vi "Init Sync Stuff.vi"(8 "error in (no error)":errorcluster, 10 "Ambient Light Bricklet in":refnum<class "Ambient Light Bricklet.lvclass">) -> (0 "error out":errorcluster, 2 "Ambient Light Bricklet out":refnum<class "Ambient Light Bricklet.lvclass">)   [LabVIEW 2011, in "Tinkerforge.lvlib" / "Ambient Light Bricklet.lvclass"]
doc: "This VI is the child implementation of \"Init Sync Stuff.vi\" and initializes all synchronization objects of this child object."
uses:
  Ambient Light Bricklet.lvclass
  Ambient Light Bricklet.lvclass/Ambient Light Bricklet.ctl
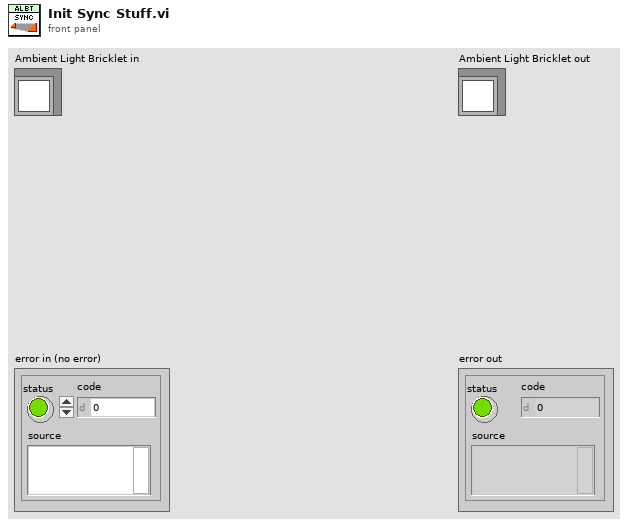
[diagram p1: front panel]
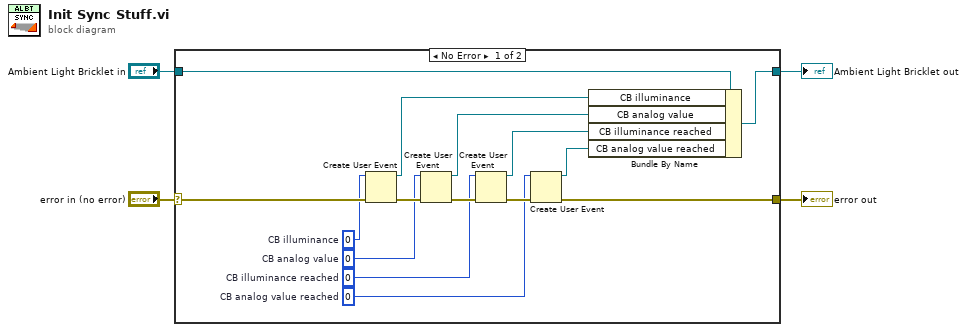
[diagram p0: block diagram]
diagram:
  n1 = case shown="No Error" "error in (no error)" {
    selector: "error in (no error)" -> [w19 w20]
    tunnel: "Ambient Light Bricklet in" -> [w10 w21]
    tunnel: [w11 w20] -> w2
    tunnel: [w9 w21] -> w1
    frame No Error {
      w12 = u16 0  # CB analog value reached
      w13 = u16 0  # CB illuminance reached
      w14 = u16 0  # CB analog value
      w18 = u16 0  # CB illuminance
      n2 = Create User Event(user event datatype=w18, error in=w19) -> (user event=w8:refnum<user-event>, error out=w17:errorcluster)
      n3 = Create User Event(user event datatype=w14, error in=w17) -> (user event=w7:refnum<user-event>, error out=w16:errorcluster)
      n4 = Create User Event(user event datatype=w13, error in=w16) -> (user event=w6:refnum<user-event>, error out=w15:errorcluster)
      n5 = Create User Event(user event datatype=w12, error in=w15) -> (user event=w5:refnum<user-event>, error out=w11:errorcluster)
      n6 = Bundle By Name(cluster=w10, "CB illuminance"=w8, "CB analog value"=w7, "CB illuminance reached"=w6, "CB analog value reached"=w5) -> (w9:refnum<class "Ambient Light Bricklet.lvclass">)
    }
    frame Error {
    }
  }
  "error out" <- w2
  "Ambient Light Bricklet out" <- w1
